vi "Minimal_FPGA.vi"() -> ()   [LabVIEW 2018]
panel:
  out "Display":i16=5
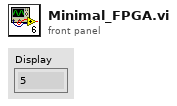
[diagram p1: front panel]
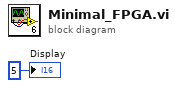
[diagram p0: block diagram]
diagram:
  "Display" <- i16 5
